vi "Set Bitmap.vi"(8 "error in (no error)":errorcluster, 10 "Bitmap":u32[][](array[numeric]), 11 "Glyph Canvas in":refnum<class "Picture Control Canvas.lvclass">) -> (0 "error out":errorcluster, 3 "Glyph Canvas out":refnum<class "Picture Control Canvas.lvclass">)   [LabVIEW 2023, in "Font Glyph Drawer Interface.lvlib" / "Picture Control Canvas.lvclass"]
uses:
  Picture Control Canvas.lvclass
  Picture Control Canvas.lvclass/Picture Control Canvas.ctl
  <vilib>/picture/picture.llb/Draw True-Color Pixmap.vi
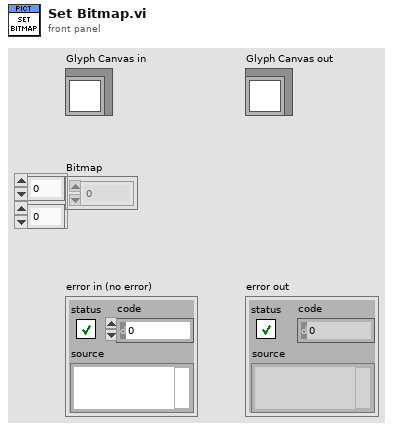
[diagram p1: front panel]
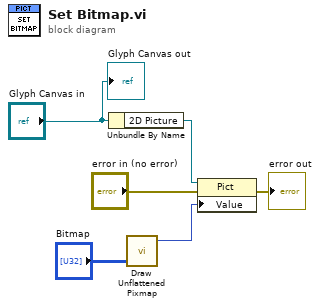
[diagram p0: block diagram]
diagram:
  n1 = Unbundle By Name("Glyph Canvas in") -> ("2D Picture"=w5:refnum<vi>)
  n2 = call-poly <vilib>:"Draw Unflattened Pixmap.vi"("data (RGB format)"="Bitmap") -> ("new picture"=w3:picture)  [unwired: 8 in]
  n3 = property class="Pict"(reference=w5, error in="error in (no error)", "Value"=w3) -> (error out=→"error out":errorcluster)  [unwired: 1 out]
  "Glyph Canvas out" <- "Glyph Canvas in"
